vi "Save File Create Backup File Path.vi"(8 "Error In":errorcluster, 10 "Station ID in":string, 11 "Tool Base Path":path) -> (0 "Error Out":errorcluster, 2 "Station ID out":string, 3 "RLT Backup Data Path":path)   [LabVIEW 2016]
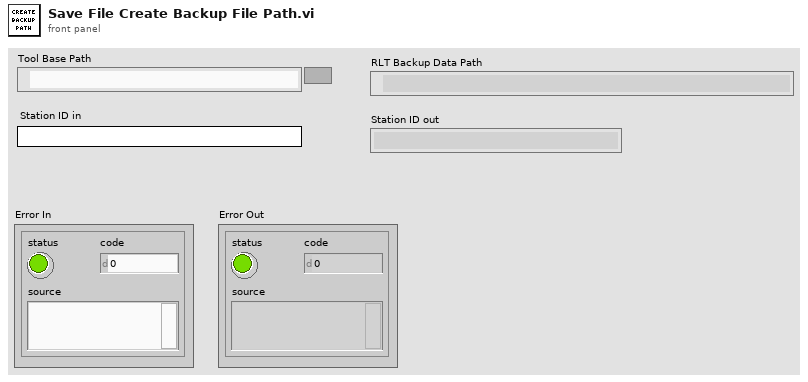
[diagram p1: front panel]
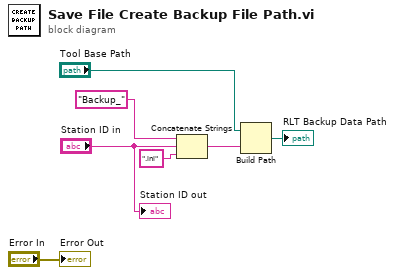
[diagram p0: block diagram]
diagram:
  n1 = Concatenate Strings("Backup_" ("name or relative path"), "Station ID in", ".ini" ("string")) -> (w5:string)
  n2 = Build Path(base path="Tool Base Path", name or relative path=w5) -> (appended path=→"RLT Backup Data Path":path)
  "Station ID out" <- "Station ID in"
  "Error Out" <- "Error In"
